vi "Stop Acquisition.vi"(8 "error in (no error)":errorcluster, 11 "Hardware Resources in":T1) -> (0 "error out":errorcluster)   [LabVIEW 2018, in "Acquisition.lvlib"]
doc: "Stops the acquisition."
uses:
  Acquisition.lvlib
  Hardware Configuration.ctl
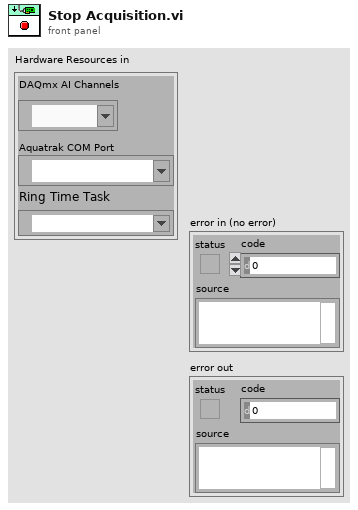
[diagram p1: front panel]
types:
  T1 = typedef "Acquisition.lvlib/Hardware Configuration.ctl" = cluster{"DAQmx AI Channels":tag, "Aquatrak COM Port":refnum<visa-resource-name>, "Ring Time Task":refnum<k21>}
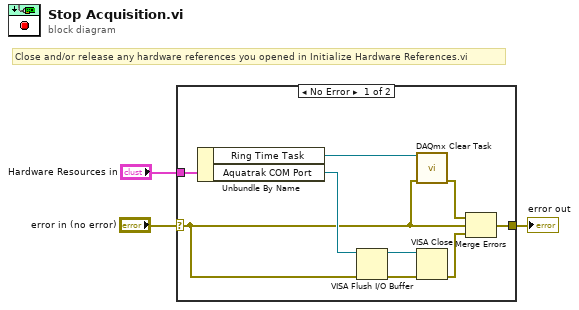
[diagram p0: block diagram]
diagram:
  # "Close and/or release any hardware references you opened in Initialize Hardware References.vi"
  n1 = case shown="No Error" "error in (no error)" {
    selector: "error in (no error)" -> [w6 w13]
    tunnel: [w12 w13] -> w2
    tunnel: "Hardware Resources in" -> [w11 _]
    frame No Error {
      n2 = Unbundle By Name(w11) -> ("Ring Time Task"=w9:refnum<k21>, "Aquatrak COM Port"=w7:refnum<visa-resource-name>)
      n3 = VISA Flush I/O Buffer(VISA resource name=w7, error in (no error)=w6) -> (VISA resource name out=w5:refnum<visa-resource-name>, error out=w4:errorcluster)  [unwired: 1 in]
      n4 = call <vilib>:"DAQmx Clear Task.vi"("task in"=w9, "error in"=w6) -> ("error out"=w10:errorcluster)  [unwired: 13 in]
      n5 = VISA Close(VISA resource name=w5, error in (no error)=w4) -> (error out=w8:errorcluster)
      n6 = Merge Errors(w10, w6, w8) -> (w12:errorcluster)
    }
    frame Error {
    }
  }
  "error out" <- w2
